vi "drive and sow.vi"   [LabVIEW 2013]
uses:
  <vilib>/myRIO/Instrument Drivers/Onboard IO/DIO/vis/Smart Open.vi
  <vilib>/myRIO/Instrument Drivers/Onboard IO/DIO/vis/Write.vi
  <vilib>/myRIO/Instrument Drivers/Onboard IO/PWM/vis/Smart Open.vi
  <vilib>/myRIO/Instrument Drivers/Onboard IO/PWM/vis/Set Duty Cycle and Frequency.vi
  <vilib>/myRIO/Common/Instrument Driver Framework/myRIO v1.0/UART/vis/myRIO v1.0 Close UART.vi
  <vilib>/myRIO/Instrument Drivers/Onboard IO/DIO/vis/Open.vi
  <vilib>/myRIO/Instrument Drivers/Onboard IO/PWM/vis/Open.vi
  <vilib>/myRIO/Common/Instrument Driver Framework/myRIO v1.0/DIO/vis/myRIO v1.1 Open DIO.vi
  <vilib>/myRIO/Common/Instrument Driver Framework/myRIO v1.0/PWM/vis/myRIO v1.1 Open PWM.vi
  <vilib>/myRIO/Common/Instrument Driver Framework/Utilities/vis/Validate Channels.vi
  <vilib>/myRIO/Common/Instrument Driver Framework/myRIO v1.0/DIO/vis/myRIO v1.0 Reserve DIO.vi
  <vilib>/myRIO/Common/Instrument Driver Framework/myRIO v1.0/PWM/vis/myRIO v1.0 Reserve PWM.vi
  <vilib>/myRIO/Common/Instrument Driver Framework/myRIO v1.0/Resource Manager/vis/myRIO v1.0 Reserve Channel List.vi
  <vilib>/myRIO/Common/Instrument Driver Framework/myRIO v1.0/DIO/vis/myRIO v1.0 Build MUX Configuration DIO.vi
  <vilib>/myRIO/Common/Instrument Driver Framework/myRIO v1.0/PWM/vis/myRIO v1.0 Build MUX Configuration PWM.vi
  <vilib>/myRIO/Common/Instrument Driver Framework/myRIO v1.0/Resource Manager/vis/myRIO v1.0 Reserve Channel.vi
  <vilib>/myRIO/Common/Instrument Driver Framework/myRIO v1.0/Resource Manager/vis/myRIO v1.0 Unreserve Channel.vi
  <vilib>/myRIO/Common/Instrument Driver Framework/myRIO v1.0/Resource Manager/vis/myRIO v1.0 Create Configuration List.vi
  <vilib>/myRIO/Common/Instrument Driver Framework/myRIO v1.0/Resource Manager/vis/myRIO v1.0 Build Mutex Name.vi
  <vilib>/myRIO/Common/Instrument Driver Framework/myRIO v1.0/myRIO v1.1 Open.vi
  <vilib>/Utility/VariantDataType/GetNumericInfo.vi
  <vilib>/Utility/error.llb/Error Cluster From Error Code.vi
  <vilib>/myRIO/Common/Instrument Driver Framework/Utilities/vis/IO Manager.vi
  <vilib>/myRIO/Common/Instrument Driver Framework/Utilities/vis/Configuration Manager.vi
  <vilib>/myRIO/Common/Instrument Driver Framework/myRIO v1.0/Resource Manager/vis/myRIO v1.0 Configure IO.vi
  <vilib>/myRIO/Common/Instrument Driver Framework/myRIO v1.0/myRIO v1.0 Close.vi
  <vilib>/myRIO/Common/Instrument Driver Framework/myRIO v1.0/DIO/vis/myRIO v1.0 Write DIO.vi
  <vilib>/myRIO/Common/Instrument Driver Framework/myRIO v1.0/PWM/vis/myRIO v1.0 Write PWM.vi
  <vilib>/myRIO/Common/Instrument Driver Framework/Utilities/vis/FPGA Ref Manager.vi
  <vilib>/myRIO/Common/Instrument Driver Framework/myRIO v1.0/myRIO v1.0 Reset FPGA.vi
  <vilib>/myRIO/Instrument Drivers/Utilities/Utilities.lvlib
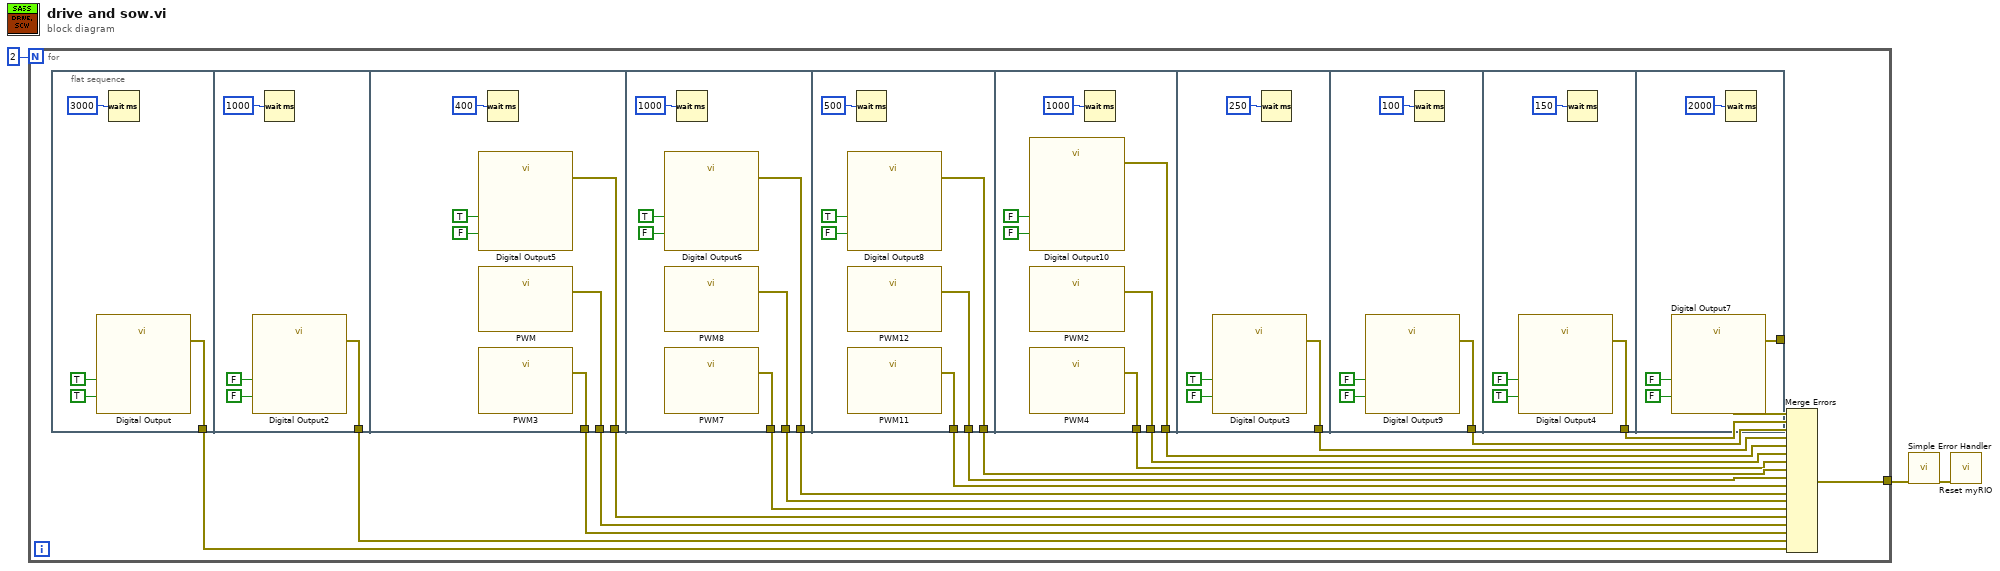
[diagram p0: block diagram]
diagram:
  n1 = for {
    N: 2 -> [_]
    tunnel: [w22] -> w2
    n2 = flat-sequence {
      tunnel: [w23] -> w21
      tunnel: [w27] -> w20
      tunnel: [w34] -> w19
      tunnel: [w35] -> w18
      tunnel: [w31] -> w17
      tunnel: [w42] -> w15
      tunnel: [w41] -> w16
      tunnel: [w37] -> w14
      tunnel: [w48] -> w13
      tunnel: [w47] -> w12
      tunnel: [w43] -> w11
      tunnel: [w53] -> w10
      tunnel: [w52] -> w9
      tunnel: [w49] -> w8
      tunnel: [w55] -> w7
      tunnel: [w59] -> w6
      tunnel: [w63] -> w5
      tunnel: [w68] -> w4
      frame #0 {
        n3 = call "Digital Output"("PWM (A/DIO0 (Pin 11))"=TRUE, "DIR (A/DIO1 (Pin 13))"=TRUE) -> ("error out"=w23:errorcluster)  [unwired: 25 in]
        n4 = Wait (ms)(milliseconds to wait=u32 3000) -> ()  [unwired: 1 out]
      }
      frame #1 {
        n5 = call "Digital Output2"("PWM (A/DIO0 (Pin 11))"=FALSE, "DIR (A/DIO1 (Pin 13))"=FALSE) -> ("error out"=w27:errorcluster)  [unwired: 25 in]
        n6 = Wait (ms)(milliseconds to wait=u32 1000) -> ()  [unwired: 1 out]
      }
      frame #2 {
        n7 = call "Digital Output5"("A/DIO5 (Pin 21)"=TRUE, "A/DIO6 (Pin 23)"=FALSE) -> ("error out"=w31:errorcluster)  [unwired: 25 in]
        n8 = call "PWM"() -> ("error out"=w35:errorcluster)  [unwired: 27 in]
        n9 = call "PWM3"() -> ("error out"=w34:errorcluster)  [unwired: 27 in]
        n10 = Wait (ms)(milliseconds to wait=u32 400) -> ()  [unwired: 1 out]
      }
      frame #3 {
        n11 = call "Digital Output6"("A/DIO5 (Pin 21)"=TRUE, "A/DIO6 (Pin 23)"=FALSE) -> ("error out"=w37:errorcluster)  [unwired: 25 in]
        n12 = call "PWM8"() -> ("error out"=w42:errorcluster)  [unwired: 27 in]
        n13 = call "PWM7"() -> ("error out"=w41:errorcluster)  [unwired: 27 in]
        n14 = Wait (ms)(milliseconds to wait=u32 1000) -> ()  [unwired: 1 out]
      }
      frame #4 {
        n15 = call "Digital Output8"("A/DIO5 (Pin 21)"=TRUE, "A/DIO6 (Pin 23)"=FALSE) -> ("error out"=w43:errorcluster)  [unwired: 25 in]
        n16 = call "PWM12"() -> ("error out"=w47:errorcluster)  [unwired: 27 in]
        n17 = call "PWM11"() -> ("error out"=w48:errorcluster)  [unwired: 27 in]
        n18 = Wait (ms)(milliseconds to wait=u32 500) -> ()  [unwired: 1 out]
      }
      frame #5 {
        n19 = call "Digital Output10"("A/DIO5 (Pin 21)"=FALSE, "A/DIO6 (Pin 23)"=FALSE) -> ("error out"=w49:errorcluster)  [unwired: 25 in]
        n20 = call "PWM2"() -> ("error out"=w52:errorcluster)  [unwired: 27 in]
        n21 = call "PWM4"() -> ("error out"=w53:errorcluster)  [unwired: 27 in]
        n22 = Wait (ms)(milliseconds to wait=u32 1000) -> ()  [unwired: 1 out]
      }
      frame #6 {
        n23 = call "Digital Output3"("A/DIO2 (Pin 15)"=TRUE, "A/DIO3 (Pin 17)"=FALSE) -> ("error out"=w55:errorcluster)  [unwired: 25 in]
        n24 = Wait (ms)(milliseconds to wait=u32 250) -> ()  [unwired: 1 out]
      }
      frame #7 {
        n25 = call "Digital Output9"("A/DIO2 (Pin 15)"=FALSE, "A/DIO3 (Pin 17)"=FALSE) -> ("error out"=w59:errorcluster)  [unwired: 25 in]
        n26 = Wait (ms)(milliseconds to wait=u32 100) -> ()  [unwired: 1 out]
      }
      frame #8 {
        n27 = call "Digital Output4"("A/DIO2 (Pin 15)"=FALSE, "A/DIO3 (Pin 17)"=TRUE) -> ("error out"=w63:errorcluster)  [unwired: 25 in]
        n28 = Wait (ms)(milliseconds to wait=u32 150) -> ()  [unwired: 1 out]
      }
      frame #9 {
        n29 = call "Digital Output7"("A/DIO2 (Pin 15)"=FALSE, "A/DIO3 (Pin 17)"=FALSE) -> ("error out"=w68:errorcluster)  [unwired: 25 in]
        n30 = Wait (ms)(milliseconds to wait=u32 2000) -> ()  [unwired: 1 out]
      }
    }
    n31 = Merge Errors(w4, w5, w6, w7, w8, w9, w10, w11, w12, w13, w14, w15, w16, w17, w18, w19, w20, w21) -> (w22:errorcluster)
  }
  n32 = call <vilib>:"Simple Error Handler.vi"("error in (no error)"=w2) -> ("error out"=w3:errorcluster)  [unwired: 4 in, 4 out]
  n33 = call <vilib>:"Reset myRIO.vi"("error in (no error)"=w3) -> ()  [unwired: 10 in, 1 out]
